vi "Write Dummy Font Class.vi"(5 "Font ref":refnum<k24>, 7 "Font":T2={"Name"="Helvetica", "Size"=12.0, "Color"=0, "Style"={"Bold"=FALSE, "Italic"=FALSE, "Underline"=FALSE, "Strikeout"=FALSE}, "Type"={"Type&direction"=enum."Select", "Embedded"=FALSE, "Encoding"=""}}, 9 "System Fonts":T1, 11 "error in (no error)":errorcluster) -> (4 "Font OUT":refnum<class "Font Class.lvclass">, 15 "error out":errorcluster)   [LabVIEW 2019, in "Font Class.lvclass"]
uses:
  <userlib>/Exaprom PDF/LV Class/Fonts Class/Font Class.lvclass
  <userlib>/Exaprom PDF/Controls/Font Controls/Font complete cluster.ctl
  <userlib>/Exaprom PDF/Controls/Font Controls/Font size.ctl
  <userlib>/Exaprom PDF/Controls/Font Controls/Font color.ctl
  <userlib>/Exaprom PDF/Controls/Font Controls/Type and encoding.ctl
  <userlib>/Exaprom PDF/Controls/Text Controls/Unicode/Type and run direction.ctl
  C:/Program Files/National Instruments/LabVIEW 2019/user.lib/Exaprom PDF/DLL/itextsharp.dll
  DLL/itextsharp.dll
  <userlib>/Exaprom PDF/Controls/Font Controls/System Fonts.ctl
  <userlib>/Exaprom PDF/LV Class/Fonts Class/Font Class.lvclass/Font Class.ctl
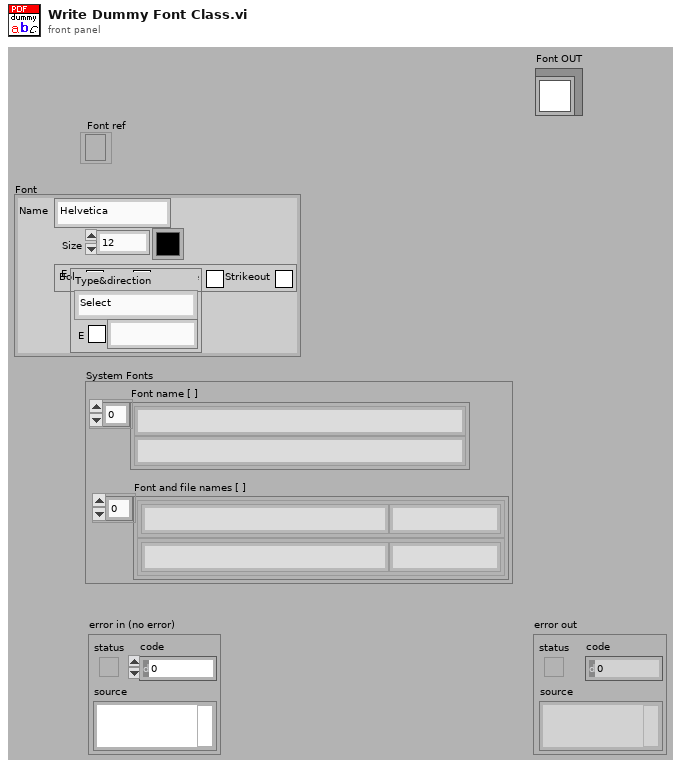
[diagram p1: front panel]
types:
  T1 = typedef "System Fonts.ctl" = cluster{"Font name [ ]":string[], "Font and file names [ ]":cluster{"Font name":string, "File name":string}[]}
  T2 = typedef "Font complete cluster.ctl" = cluster{"Name":string, "Size":T3, "Color":T4, "Style":cluster{"Bold":bool, "Italic":bool, "Underline":bool, "Strikeout":bool}, "Type":T5}
  T3 = typedef "Font size.ctl" = sgl
  T4 = typedef "Font color.ctl" = u32
  T5 = typedef "Type and encoding.ctl" = cluster{"Type&direction":T6, "Embedded":bool, "Encoding":string}
  T6 = typedef "Type and run direction.ctl" = enum16{"Select", "ASCII", "UTF-16", "UTF-16 (default)", "UTF-16 (LTR)", "UTF-16 (RTL)"}
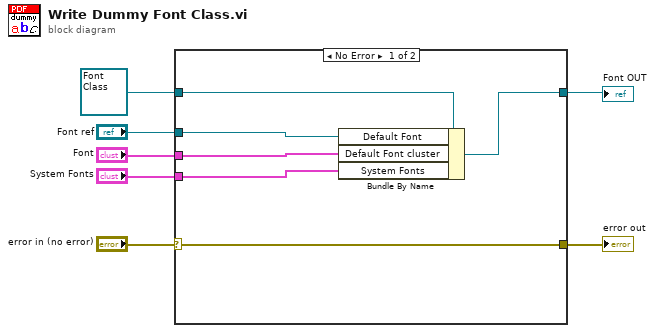
[diagram p0: block diagram]
diagram:
  n1 = case shown="No Error" "error in (no error)" {
    selector: "error in (no error)" -> [w11 w15]
    tunnel: [w11 w15] -> w6
    tunnel: [w13 w14] -> w5
    tunnel: refnum<class "Font Class.lvclass"> refnum ("Font IN") -> [w12 w14]
    tunnel: "Font ref" -> [w10 _]
    tunnel: "Font" -> [w9 _]
    tunnel: "System Fonts" -> [w8 _]
    frame No Error {
      n2 = Bundle By Name(cluster=w12, "Default Font"=w10, "Default Font cluster"=w9, "System Fonts"=w8) -> (w13:refnum<class "Font Class.lvclass">)
    }
    frame Error {
    }
  }
  "error out" <- w6
  "Font OUT" <- w5
